vi "c_GENERATE_OPERATIONS.vi"(11 "FiringOrder":refnum<vi>[](array[refnum])) -> (3 "Array":refnum<class "CodeElement.lvclass">[](array[class]))   [LabVIEW 2017]
uses:
  CodeElements/Base/CodeElement.lvclass
  CodeElements/RawCodeElement_class/RawCodeElement.lvclass
  E:/Code_Generator/CodeElements/Base/CodeElement.lvclass
  CodeElements/Typedef_Element_class/Typedef_Element.lvclass
  CodeElements/SwitchCaseElement_class/SwitchCaseElement.lvclass
  CodeElements/SetIntermediateValueDoLast_class/SetIntermediateValueDoLast.lvclass
  CodeElements/SetIntermediateValue_class/SetIntermediateValue.lvclass
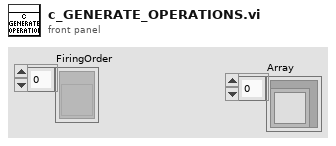
[diagram p1: front panel]
types:
  T1 = cluster{"Array":refnum<class "CodeElement.lvclass">[]}
  T2 = cluster{"CodeElements":refnum<class "CodeElement.lvclass">[]}
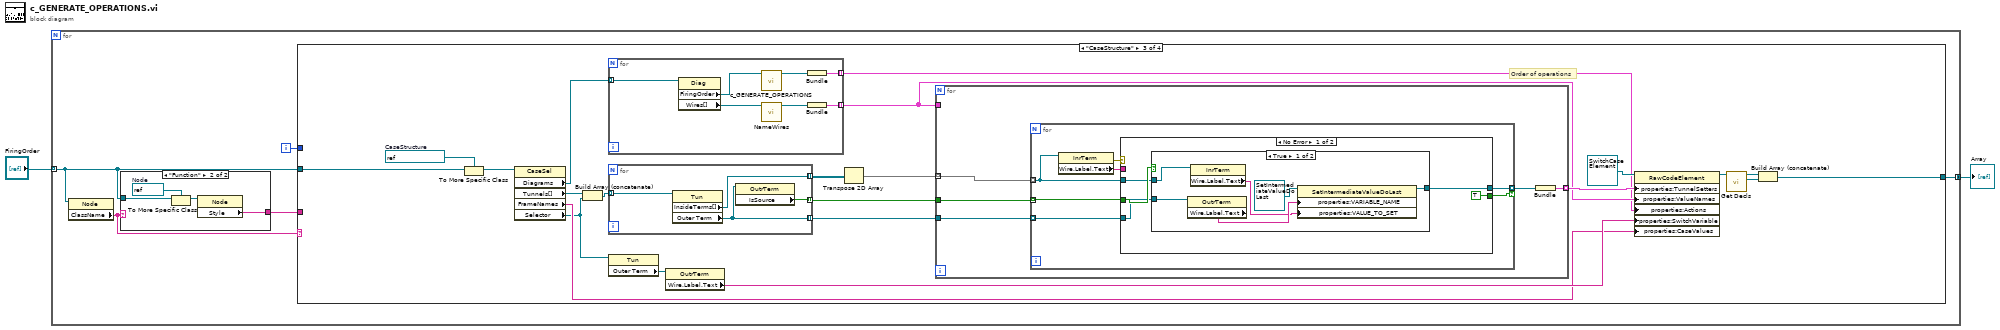
[diagram p0: block diagram]
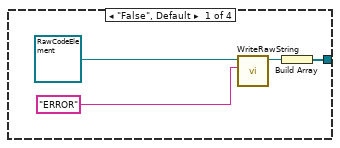
[diagram p2: hidden frame]
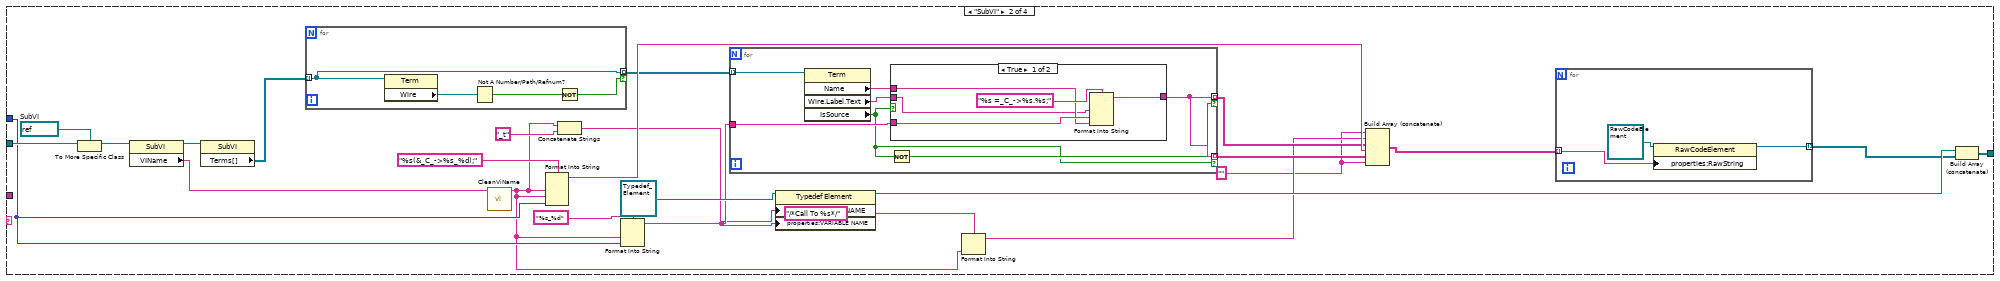
[diagram p3: hidden frame]
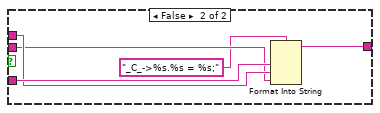
[diagram p4: hidden frame]
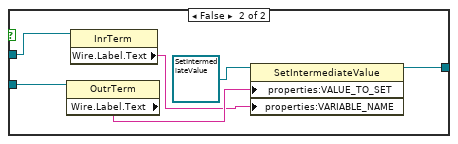
[diagram p5: hidden frame]
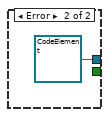
[diagram p6: hidden frame]
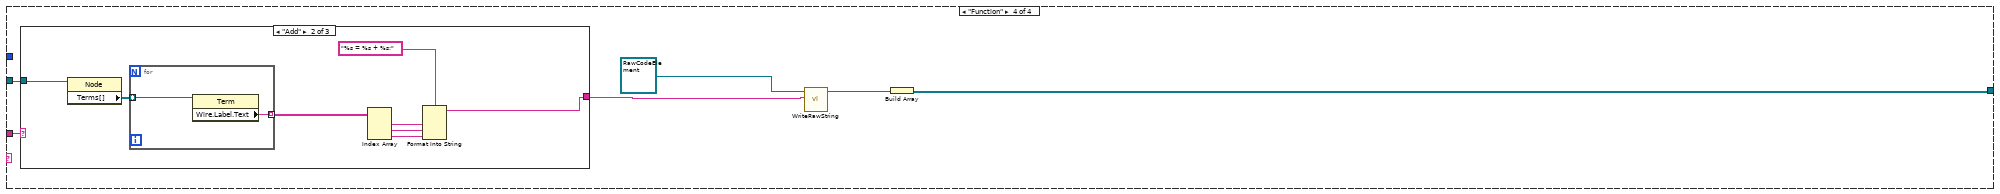
[diagram p7: hidden frame]
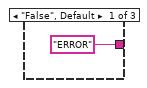
[diagram p8: hidden frame]
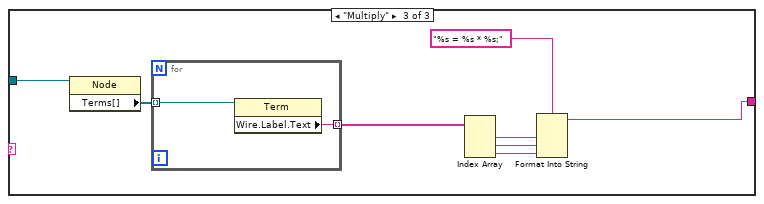
[diagram p9: hidden frame]
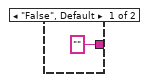
[diagram p10: hidden frame]
diagram:
  n1 = for {
    tunnel: "FiringOrder" -> [w5] mode=indexing
    tunnel: [w4] -> w1 mode=concatenating
    i -> [w3]
    n2 = property class="Node"(reference=w5) -> ("ClassName"=w7:string)  [unwired: 1 in, 2 out]
    n3 = case shown="\"Function\"" w7 {
      tunnel: w5 -> [_ w155]
      tunnel: ["" ("Desc") w152] -> w6
      frame "False", Default {
      }
      frame "Function" {
        w154 = refnum<vi> refnum  # Node
        n4 = To More Specific Class(target class=w154, reference=w155) -> (specific class reference=w153:refnum<vi>)  [unwired: 1 in, 1 out]
        n5 = property class="Node"(reference=w153) -> ("Style"=w152:string)  [unwired: 1 in, 2 out]
      }
    }
    n6 = case shown="\"CaseStructure\"" w7 {
      tunnel: w6 -> [_ _ _ w129]
      tunnel: w5 -> [_ w36 w82 w128]
      tunnel: [w9 w19 w72 w124] -> w4
      tunnel: w3 -> [_ w29 _ _]
      frame "False", Default {
        n7 = call-dynamic "WriteRawString.vi"("RawString"="ERROR", "object in"=refnum<class "RawCodeElement.lvclass"> refnum) -> ("object out"=w10:refnum<class "RawCodeElement.lvclass">)  [unwired: 8 in, 1 out]
        n8 = Build Array(w10) -> (w9:refnum<class "RawCodeElement.lvclass">[])
      }
      frame "SubVI" {
        w12 = ""
        w35 = refnum<vi> refnum  # SubVI
        n9 = To More Specific Class(target class=w35, reference=w36) -> (specific class reference=w34:refnum<vi>)  [unwired: 1 in, 1 out]
        n10 = property class="SubVI"(reference=w34) -> (reference out=w28:refnum<vi>, "VIName"=w33:string)  [unwired: 1 in, 1 out]
        n11 = property class="SubVI"(reference=w28) -> ("Terms[]"=w25:refnum<vi>[])  [unwired: 1 in, 2 out]
        n12 = for {
          tunnel: w25 -> [w43] mode=indexing
          tunnel: [w43] -> w24 mode=indexing if=w40
          n13 = property class="Term"(reference=w43) -> ("Wire"=w42:refnum<vi>)  [unwired: 1 in, 2 out]
          n14 = Not A Number/Path/Refnum?(number/path/refnum=w42) -> (NaN/Path/Refnum?=w41:bool)
          n15 = Not(x=w41) -> (.not. x?=w40:bool)
        }
        n16 = call "CleanViName.vi"("Name"=w33) -> ("submatch 1"=w14:string)  [unwired: 10 in]
        n17 = Format Into String(format string="%s(&_C_->%s_%d);", w14, w14, w29) -> (resulting string=w31:string)  [unwired: 2 in, 1 out]
        n18 = Concatenate Strings(w14, "_t" ("string")) -> (w18:string)
        n19 = Format Into String(format string="%s_%d", w14, w29) -> (resulting string=w22:string)  [unwired: 2 in, 1 out]
        n20 = for {
          tunnel: w24 -> [w50] mode=indexing
          tunnel: w22 -> [w49]
          tunnel: [w46] -> w27 mode=indexing if=w45
          tunnel: [w46] -> w26 mode=indexing if=w44
          n21 = property class="Term"(reference=w50) -> ("Name"=w48:string, "Wire.Label.Text"=w47:string, "IsSource"=w44:bool)  [unwired: 1 in, 2 out]
          n22 = Not(x=w44) -> (.not. x?=w45:bool)
          n23 = case shown="True" w44 {
            tunnel: w49 -> [w53 w60]
            tunnel: w48 -> [w52 w59]
            tunnel: w47 -> [w51 w58]
            tunnel: [w55 w57] -> w46
            frame True {
              n24 = Format Into String(format string="%s =_C_->%s.%s;", w51, w53, w52) -> (resulting string=w55:string)  [unwired: 2 in, 1 out]
            }
            frame False {
              n25 = Format Into String(format string="_C_->%s.%s = %s;", w60, w59, w58) -> (resulting string=w57:string)  [unwired: 2 in, 1 out]
            }
          }
        }
        n26 = property class="Typedef Element"(reference=refnum<class "Typedef_Element.lvclass"> refnum ("Typedef Element"), "properties:TYPE NAME"=w18, "properties:VARIABLE NAME"=w22) -> (reference out=w21:refnum<class "Typedef_Element.lvclass">)  [unwired: 1 in, 1 out]
        n27 = Format Into String(format string="/*Call To %s*/", w14) -> (resulting string=w13:string)  [unwired: 2 in, 1 out]
        n28 = Build Array (concatenate)(w12, w13, w27, w31, w26, w12) -> (w16:string[])
        n29 = for {
          tunnel: [w39] -> w20 mode=indexing
          tunnel: w16 -> [w37] mode=indexing
          n30 = property class="RawCodeElement"(reference=refnum<class "RawCodeElement.lvclass"> refnum ("RawCodeElement.lvclass"), "properties:RawString"=w37) -> (reference out=w39:refnum<class "RawCodeElement.lvclass">)  [unwired: 1 in, 1 out]
        }
        n31 = Build Array (concatenate)(w21, w20) -> (w19:refnum<class "CodeElement.lvclass">[])
      }
      frame "CaseStructure" {
        w81 = refnum<vi> refnum  # CaseStructure
        # "Order of operations"
        n32 = To More Specific Class(target class=w81, reference=w82) -> (specific class reference=w80:refnum<vi>)  [unwired: 1 in, 1 out]
        n33 = property class="CaseSel"(reference=w80) -> ("Diagrams"=w79:refnum<vi>[], "Tunnels[]"=w70:refnum<vi>[], "FrameNames"=w71:string[], "Selector"=w63:refnum<vi>)  [unwired: 1 in, 2 out]
        n34 = Build Array (concatenate)(w70, w63) -> (w64:refnum<vi>[])
        n35 = for {
          tunnel: w79 -> [w123] mode=indexing
          tunnel: [w119] -> w75 mode=indexing
          tunnel: [w117] -> w74 mode=indexing
          n36 = property class="Diag"(reference=w123) -> ("FiringOrder"=w122:refnum<vi>[], "Wires[]"=w121:refnum<vi>[])  [unwired: 1 in, 2 out]
          n37 = call "c_GENERATE_OPERATIONS.vi"("FiringOrder"=w122) -> ("Array"=w118:refnum<class "CodeElement.lvclass">[])  [unwired: 10 in]
          n38 = call "NameWires.vi"("Wires[]"=w121) -> ("CodeElements"=w120:refnum<class "CodeElement.lvclass">[])  [unwired: 10 in]
          n39 = Bundle("Array"=w118) -> (w117:T1)  [unwired: 1 in]
          n40 = Bundle("CodeElements"=w120) -> (w119:T2)  [unwired: 1 in]
        }
        n41 = for {
          tunnel: w64 -> [w86] mode=indexing
          tunnel: [w85] -> w69 mode=indexing
          tunnel: [w84] -> w68 mode=indexing
          tunnel: [w83] -> w62 mode=indexing
          n42 = property class="Tun"(reference=w86) -> ("InsideTerms[]"=w83:refnum<vi>[], "Outer Term"=w85:refnum<vi>)  [unwired: 1 in, 2 out]
          n43 = property class="OutrTerm"(reference=w85) -> ("IsSource"=w84:bool)  [unwired: 1 in, 2 out]
        }
        n44 = property class="Tun"(reference=w63) -> ("Outer Term"=w78:refnum<vi>)  [unwired: 1 in, 2 out]
        n45 = property class="OutrTerm"(reference=w78) -> ("Wire.Label.Text"=w73:string)  [unwired: 1 in, 2 out]
        n46 = Transpose 2D Array(2D array=w62) -> (transposed array=w61:refnum<vi>[][])
        n47 = for {
          tunnel: [w91] -> w76 mode=indexing
          tunnel: w75 -> [_]
          tunnel: w69 -> [w89]
          tunnel: w68 -> [w90]
          tunnel: w61 -> [w87] mode=indexing
          n48 = for {
            tunnel: w90 -> [w98] mode=indexing
            tunnel: w89 -> [w97] mode=indexing
            tunnel: w87 -> [w94] mode=indexing
            tunnel: [w96] -> w88 mode=indexing if=w95
            n49 = property class="InrTerm"(reference=w94) -> (error out=w93:errorcluster, "Wire.Label.Text"=w92:string)  [unwired: 1 in, 1 out]
            n50 = case shown="No Error" w93 {
              tunnel: w98 -> [w103 _]
              tunnel: w97 -> [w102 _]
              tunnel: [w101 refnum<class "CodeElement.lvclass"> refnum ("SetReturnValue")] -> w96
              tunnel: w94 -> [w100 _]
              tunnel: [TRUE _] -> w95
              tunnel: w92 -> [_ _]
              frame No Error {
                n51 = case shown="True" w103 {
                  tunnel: w102 -> [w107 w112]
                  tunnel: w100 -> [w108 w111]
                  tunnel: [w106 w114] -> w101
                  frame True {
                    n52 = property class="OutrTerm"(reference=w107) -> ("Wire.Label.Text"=w105:string)  [unwired: 1 in, 2 out]
                    n53 = property class="InrTerm"(reference=w108) -> ("Wire.Label.Text"=w104:string)  [unwired: 1 in, 2 out]
                    n54 = property class="SetIntermediateValueDoLast"(reference=refnum<class "SetIntermediateValueDoLast.lvclass"> refnum ("SetIntermediateValueDoLast"), "properties:VARIABLE_NAME"=w105, "properties:VALUE_TO_SET"=w104) -> (reference out=w106:refnum<class "SetIntermediateValueDoLast.lvclass">)  [unwired: 1 in, 1 out]
                  }
                  frame False {
                    n55 = property class="OutrTerm"(reference=w112) -> ("Wire.Label.Text"=w113:string)  [unwired: 1 in, 2 out]
                    n56 = property class="InrTerm"(reference=w111) -> ("Wire.Label.Text"=w110:string)  [unwired: 1 in, 2 out]
                    n57 = property class="SetIntermediateValue"(reference=refnum<class "SetIntermediateValue.lvclass"> refnum ("SetReturnValue"), "properties:VALUE_TO_SET"=w113, "properties:VARIABLE_NAME"=w110) -> (reference out=w114:refnum<class "SetIntermediateValue.lvclass">)  [unwired: 1 in, 1 out]
                  }
                }
              }
              frame Error {
              }
            }
          }
          n58 = Bundle(w88) -> (w91:cluster{refnum<class "CodeElement.lvclass">[]})  [unwired: 1 in]
        }
        n59 = property class="RawCodeElement"(reference=refnum<class "SwitchCaseElement.lvclass"> refnum ("RawCodeElement"), "properties:TunnelSetters"=w76, "properties:ValueNames"=w75, "properties:Actions"=w74, "properties:SwitchVariable"=w73, "properties:CaseValues"=w71) -> (reference out=w67:refnum<class "SwitchCaseElement.lvclass">)  [unwired: 1 in, 1 out]
        n60 = call-dynamic "Get Decls.vi"("object in"=w67) -> ("Declarations"=w65:refnum<class "CodeElement.lvclass">[], "object out"=w66:refnum<class "SwitchCaseElement.lvclass">)  [unwired: 8 in, 1 out]
        n61 = Build Array (concatenate)(w66, w65) -> (w72:refnum<class "CodeElement.lvclass">[])
      }
      frame "Function" {
        n62 = case shown="\"Add\"" w129 {
          tunnel: w128 -> [_ w138 w148]
          tunnel: ["ERROR" w131 w141] -> w126
          frame "False", Default {
          }
          frame "Add" {
            n63 = property class="Node"(reference=w138) -> ("Terms[]"=w137:refnum<vi>[])  [unwired: 1 in, 2 out]
            n64 = for {
              tunnel: w137 -> [w140] mode=indexing
              tunnel: [w139] -> w136 mode=indexing
              n65 = property class="Term"(reference=w140) -> ("Wire.Label.Text"=w139:string)  [unwired: 1 in, 2 out]
            }
            n66 = Index Array(array=w136) -> (element #1=w134:string, element #2=w133:string, element #3=w132:string)  [unwired: 3 in]
            n67 = Format Into String(format string="%s = %s + %s;", w134, w133, w132) -> (resulting string=w131:string)  [unwired: 2 in, 1 out]
          }
          frame "Multiply" {
            n68 = property class="Node"(reference=w148) -> ("Terms[]"=w147:refnum<vi>[])  [unwired: 1 in, 2 out]
            n69 = for {
              tunnel: w147 -> [w150] mode=indexing
              tunnel: [w149] -> w146 mode=indexing
              n70 = property class="Term"(reference=w150) -> ("Wire.Label.Text"=w149:string)  [unwired: 1 in, 2 out]
            }
            n71 = Index Array(array=w146) -> (element #1=w144:string, element #2=w143:string, element #3=w142:string)  [unwired: 3 in]
            n72 = Format Into String(format string="%s = %s * %s;", w144, w143, w142) -> (resulting string=w141:string)  [unwired: 2 in, 1 out]
          }
        }
        n73 = call-dynamic "WriteRawString.vi"("RawString"=w126, "object in"=refnum<class "RawCodeElement.lvclass"> refnum ("RawCodeElement.lvclass")) -> ("object out"=w125:refnum<class "RawCodeElement.lvclass">)  [unwired: 8 in, 1 out]
        n74 = Build Array(w125) -> (w124:refnum<class "RawCodeElement.lvclass">[])
      }
    }
  }
  "Array" <- w1
